vi "XXPathPlanner_ConstraintsZone_ForSegmentIndex.vi"(9 "SegmentIndex":i32, 11 "ConstraintsZone":T1={"minPosition"=0.0, "maxPosition"=0.0, "Constraints"={"MaxVelocityMps;"=0.0, "MaxAccelerationMpsSq;"=0.0, "MaxAngularVelRadPsEc;"=0.0, "MaxAngularAccRadPSecSq"=0.0, "Exists"=FALSE, "Unlimited"=FALSE, "NominalVoltageVolts"=12.0}, "Present"=FALSE}) -> (3 "new Constraints Zone":T1={"minPosition"=0.0, "maxPosition"=0.0, "Constraints"={"MaxVelocityMps;"=0.0, "MaxAccelerationMpsSq;"=0.0, "MaxAngularVelRadPsEc;"=0.0, "MaxAngularAccRadPSecSq"=0.0, "Exists"=FALSE, "Unlimited"=FALSE, "NominalVoltageVolts"=12.0}, "Present"=FALSE})   [LabVIEW 2019]
doc: "Transform the positions of this zone for a given segment number.\n \nFor example, a zone from [1.5, 2.0] for the segment 1 will have the positions [0.5, 1.0]\n \nInputs: \n -- ConstraintsZone - cluster - definition of zone\n -- segmentIndex - int - The segment index to transform positions for\n\nOutputs:\n -- NewConstraintsZone - cluster - The transformed zone"
uses:
  TypeDef/PathPlannerConstraintsZone.ctl
  TypeDef/PathPlannerPathConstraints.ctl
  PathPlanner24.lvlib
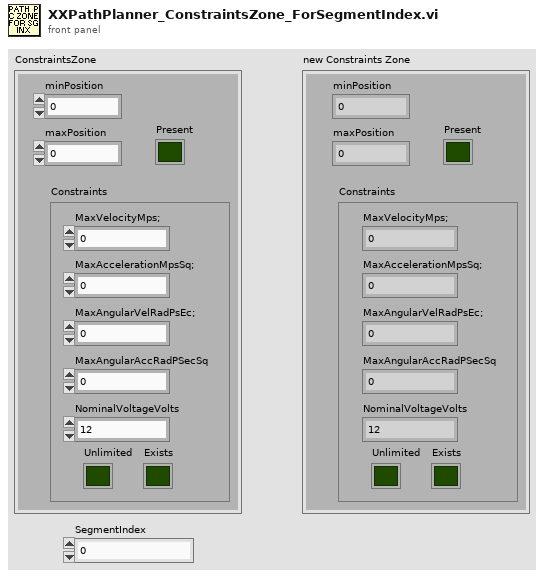
[diagram p1: front panel]
types:
  T1 = typedef "PathPlanner24.lvlib/PathPlannerConstraintsZone.ctl" = cluster{"minPosition":dbl, "maxPosition":dbl, "Constraints":T2, "Present":bool}
  T2 = typedef "PathPlanner24.lvlib/PathPlannerPathConstraints.ctl" = cluster{"MaxVelocityMps;":dbl, "MaxAccelerationMpsSq;":dbl, "MaxAngularVelRadPsEc;":dbl, "MaxAngularAccRadPSecSq":dbl, "Exists":bool, "Unlimited":bool, "NominalVoltageVolts":dbl}
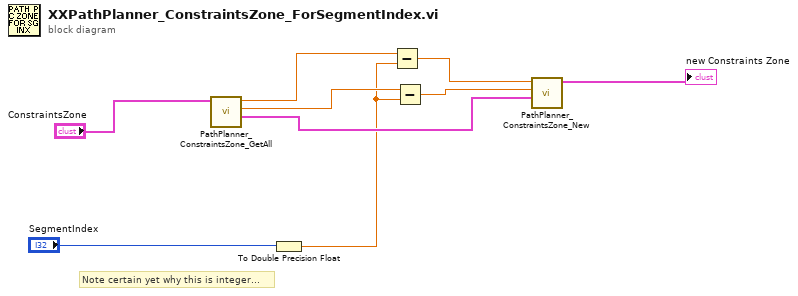
[diagram p0: block diagram]
diagram:
  # "Note certain yet why this is integer..."
  n1 = call "PathPlanner_ConstraintsZone_GetAll.vi"("ConstraintsZone"="ConstraintsZone") -> ("Constraints"=w6:T2, "maxWaypointPos"=w3:dbl, "minWaypointPos"=w7:dbl)  [unwired: 8 in]
  n2 = To Double Precision Float(number="SegmentIndex") -> (double precision float=w1:dbl)
  n3 = Subtract(x=w7, y=w1) -> (x-y=w5:dbl)
  n4 = Subtract(x=w3, y=w1) -> (x-y=w2:dbl)
  n5 = call "PathPlanner_ConstraintsZone_New.vi"("Constraints"=w6, "maxPosition"=w2, "minPosition"=w5) -> ("ConstraintsZone"=→"new Constraints Zone":T1)  [unwired: 8 in]
